vi "MainPC.vi"() -> ()   [LabVIEW 2017]
doc: "Use this template to build a simple state machine design pattern. Each state executes code and determines which state to transition to."
uses:
  Projekt-RubikLibrary/ServoEnumControl.ctl
  Projekt-RubikLibrary/ServoCCWControl.ctl
  TypeDefs/UIState.ctl
  TypeDefs/CommandsRT.ctl
  Projekt-RubikLibrary/RubikLibrary.lvlib
panel:
  out "Grip State":bool[](array[boolean])
  in  "Gripper":bool
  in  "Turn by":T1
  in  "Servo/Gripper":T2
  in  "Turn Button":bool
  in  "Exit":bool
  # "Rubik's Cube Move&Grip"
  # "Turn Servo by +/-90°\nOpen/close gripper, select Left/Front/Right gripper\n\nStates of all grippers are shown"
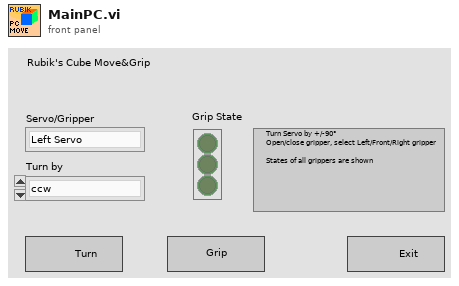
[diagram p1: front panel]
types:
  T1 = typedef "RubikLibrary.lvlib/ServoCCWControl.ctl" = enum16{"ccw", "cw"}
  T2 = typedef "RubikLibrary.lvlib/ServoEnumControl.ctl" = enum16{"Left Servo", "Front Servo", "Right Servo"}
  T3 = typedef "UIState.ctl" = enum16{"Wait for Event", "Initializing", "Turning", "Gripping", "Exiting"}
  T4 = typedef "CommandsRT.ctl" = enum16{"Initialize", "Turn", "Grip", "Exit"}
  T5 = typedef "DataStreamCluster.ctl" = cluster{"Commands":T4, "Variant":variant}
  T6 = cluster{"Servo/Gripper ":T2, "Turn by":T1, "Gripper":bool}
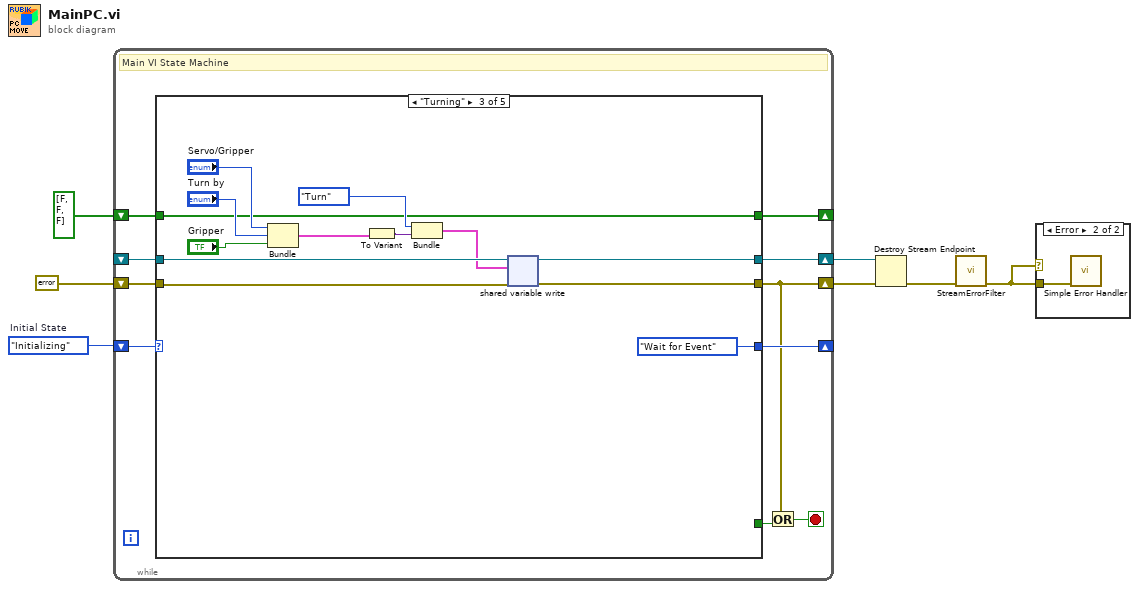
[diagram p0: block diagram]
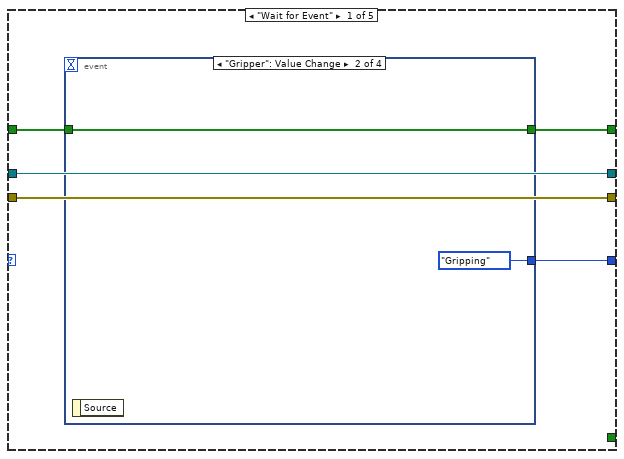
[diagram p3: hidden frame]
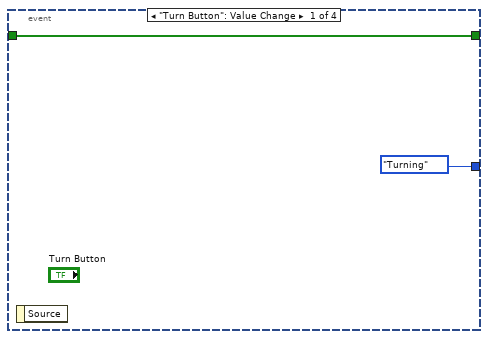
[diagram p4: hidden frame]
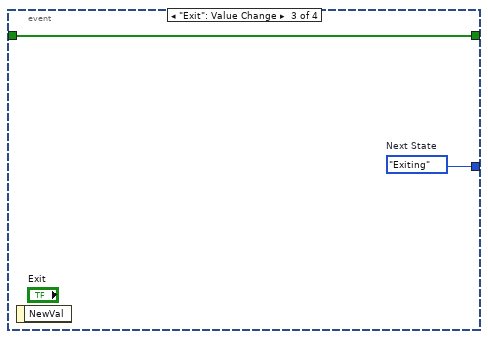
[diagram p5: hidden frame]
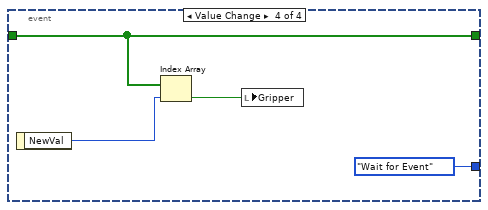
[diagram p6: hidden frame]
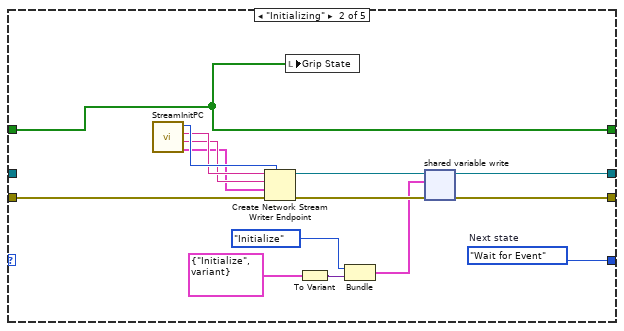
[diagram p7: hidden frame]
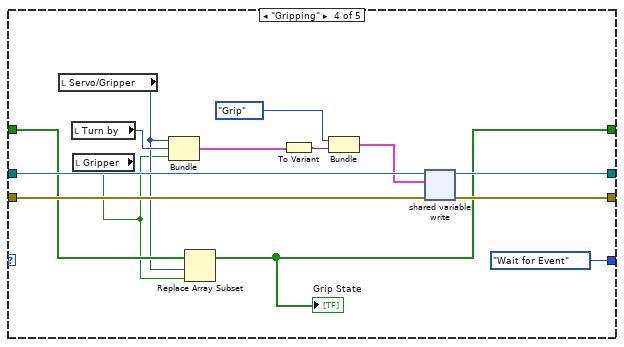
[diagram p8: hidden frame]
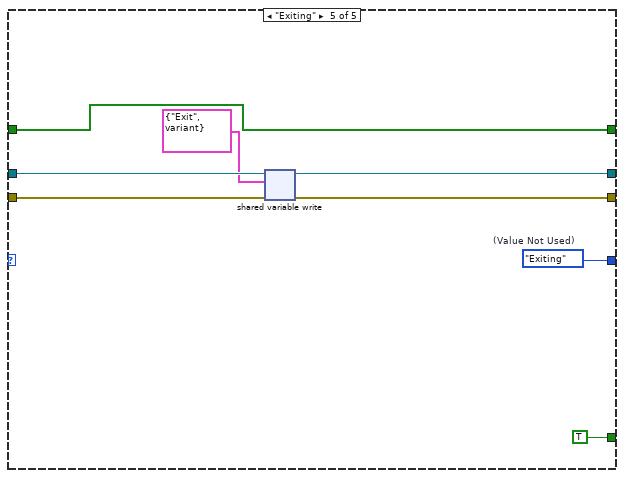
[diagram p9: hidden frame]
diagram:
  w7 = UIState."Initializing"  # Initial State
  n1 = while {
    shift-right: [w17] -> _
    shift-left: w7 -> [w14]
    shift-right: [w10] -> w5
    shift-left: errorcluster {"status"=FALSE, "code"=0, "source"=""} ("error constant") -> [w13]
    shift-right: [w12] -> w4
    shift-left: _ -> [w11]
    shift-right: [w8] -> _
    shift-left: bool[] [FALSE, FALSE, FALSE] ("Grip State") -> [w9]
    stop <- w15 stop-if-true
    # "Main VI State Machine"
    n2 = case shown="\"Turning\"" w14 {
      tunnel: [w22 w47 UIState."Wait for Event" ("(Value Not Used)") UIState."Wait for Event" ("(Value Not Used)") w82] -> w17
      tunnel: [_ _ _ _ TRUE ("Stop Loop?")] -> w16
      tunnel: [w20 w37 w58 w69 w79] -> w10
      tunnel: w13 -> [w20 w43 w59 w70 w80]
      tunnel: [w21 w35 w57 w68 w78] -> w12
      tunnel: w11 -> [w21 _ w56 w71 w77]
      tunnel: w9 -> [w19 w41 w48 w64 w75]
      tunnel: [w18 w41 w48 w61 w75] -> w8
      frame "Wait for Event" {
        # "Wait for Event - Use an Event Structure to monitor the user interface for events that run different states of the state machine."
        n3 = event shown="[1] \"Gripper\": Value Change" {
          selector: _ -> [_ _ _ _]
          dyn-events: _ -> [_ _ _ _]
          timeout: _ -> [_ _ _ _]
          tunnel: [UIState."Turning" ("Next State") UIState."Gripping" ("Next State") w28 UIState."Wait for Event" ("Next State")] -> w22
          tunnel: w19 -> [w23 w25 w27 w31]
          tunnel: [w23 w25 w27 w31] -> w18
          event "Turn Button": Value Change {
            n4 = event-data() -> ()  [unwired: 1 in, 1 out]
          }
          event "Gripper": Value Change {
            n5 = event-data() -> ()  [unwired: 1 in, 1 out]
          }
          event "Exit": Value Change {
            w28 = UIState."Exiting"  # Next State
            n6 = event-data() -> ()  [unwired: 1 in, 1 out]
          }
          event Value Change {
            n7 = event-data() -> ("NewVal"=w32:T2)  [unwired: 1 in]
            n8 = Index Array(array=w31, index=w32) -> (element=w30:bool)
            n9 = local write "Gripper"(w30) -> ()
          }
        }
      }
      frame "Initializing" {
        w47 = UIState."Wait for Event"  # Next state
        # "Initialize - Initialize the application."
        n10 = call "StreamInitPC.vi"() -> ("data cluster"=w42:T5, "reader name"=w44:string, "writer name"=w45:string, "writer buffer size"=w46:i32)  [unwired: 4 in]
        n11 = Create Network Stream Writer Endpoint(7:w46, 8:w43, 9:w42, 10:w44, 11:w45) -> (0:w38:errorcluster, 3:w36:refnum<k21>)  [unwired: 2 in]
        n12 = local write "Grip State"(w41) -> ()
        n13 = To Variant(anything=cluster{"Commands":T4, variant} {"Commands"=enum."Initialize", variant}) -> (Variant=w39:variant)
        n14 = Bundle("Commands"=CommandsRT."Initialize", "Variant"=w39) -> (w34:cluster{"Commands":T4, "Variant":variant})  [unwired: 1 in]
        n15 = shared-variable-write(w36, w38, w34) -> (w35:refnum<k21>, w37:errorcluster)  [unwired: 1 in, 1 out]
      }
      frame "Turning" {
        n16 = Bundle("Servo/Gripper"="Servo/Gripper", "Turn by"="Turn by", "Gripper"="Gripper") -> (w51:T6)  [unwired: 1 in]
        n17 = To Variant(anything=w51) -> (Variant=w54:variant)
        n18 = Bundle("Commands"=CommandsRT."Turn", "Variant"=w54) -> (w49:cluster{"Commands":T4, "Variant":variant})  [unwired: 1 in]
        n19 = shared-variable-write(w56, w59, w49) -> (w57:refnum<k21>, w58:errorcluster)  [unwired: 1 in, 1 out]
      }
      frame "Gripping" {
        n20 = local read "Servo/Gripper"() -> (w63:T2)
        n21 = local read "Turn by"() -> (w66:T1)
        n22 = local read "Gripper"() -> (w62:bool)
        n23 = Bundle("Servo/Gripper"=w63, "Turn by"=w66, "Gripper"=w62) -> (w72:T6)  [unwired: 1 in]
        n24 = Replace Array Subset(array=w64, new element=w62, index=w63) -> (w61:bool[])
        "Grip State" <- w61
        n25 = To Variant(anything=w72) -> (Variant=w73:variant)
        n26 = Bundle("Commands"=CommandsRT."Grip", "Variant"=w73) -> (w65:cluster{"Commands":T4, "Variant":variant})  [unwired: 1 in]
        n27 = shared-variable-write(w71, w70, w65) -> (w68:refnum<k21>, w69:errorcluster)  [unwired: 1 in, 1 out]
      }
      frame "Exiting" {
        w82 = UIState."Exiting"  # (Value Not Used)
        n28 = shared-variable-write(w77, w80, cluster{"Commands":T4, variant} {"Commands"=enum."Exit", variant} ("anything")) -> (w78:refnum<k21>, w79:errorcluster)  [unwired: 1 in, 1 out]
      }
    }
    n29 = Or(x=w10, y=w16) -> (x .or. y?=w15:bool)
  }
  n30 = Destroy Stream Endpoint(8:w5, 11:w4) -> (0:w6:errorcluster)
  n31 = call "StreamErrorFilter.vi"("error in (no error)"=w6) -> ("error out"=w2:errorcluster)  [unwired: 10 in]
  n32 = case shown="Error" w2 {
    tunnel: w2 -> [_ w83]
    frame No Error {
    }
    frame Error {
      n33 = call <vilib>:"Simple Error Handler.vi"("error in (no error)"=w83) -> ()  [unwired: 4 in, 5 out]
    }
  }
